vi "Ex6_Principal.vi"() -> ()   [LabVIEW 2019]
uses:
  Ex6_Secondaire.vi
panel:
  in  "stop":bool
  out "2D Picture":picture
  out "Max":i16
  out "Tentatives":i16
  in  "Ouvrir":bool
  out "Boolean 2":bool
  out "Boolean":bool
  in  "Knob 3":i8(knob) scale=0.0..9.0
  in  "Knob 2":i8(knob) scale=0.0..9.0
  in  "Knob":i16(knob) scale=0.0..9.0
  # "/"
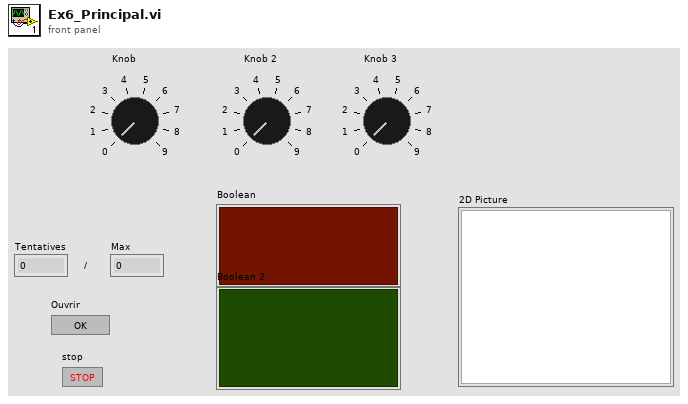
[diagram p1: front panel]
types:
  T1 = enum8{"Enabled", "Disabled", "Disabled and Grayed Out"}
  T2 = typedef "imagedata.ctl" = cluster{"image type":i32, "image depth":i32, "image":u8[], "mask":u8[], "colors":u32[], "Rectangle":cluster{"left":i16, "top":i16, "right":i16, "bottom":i16}}
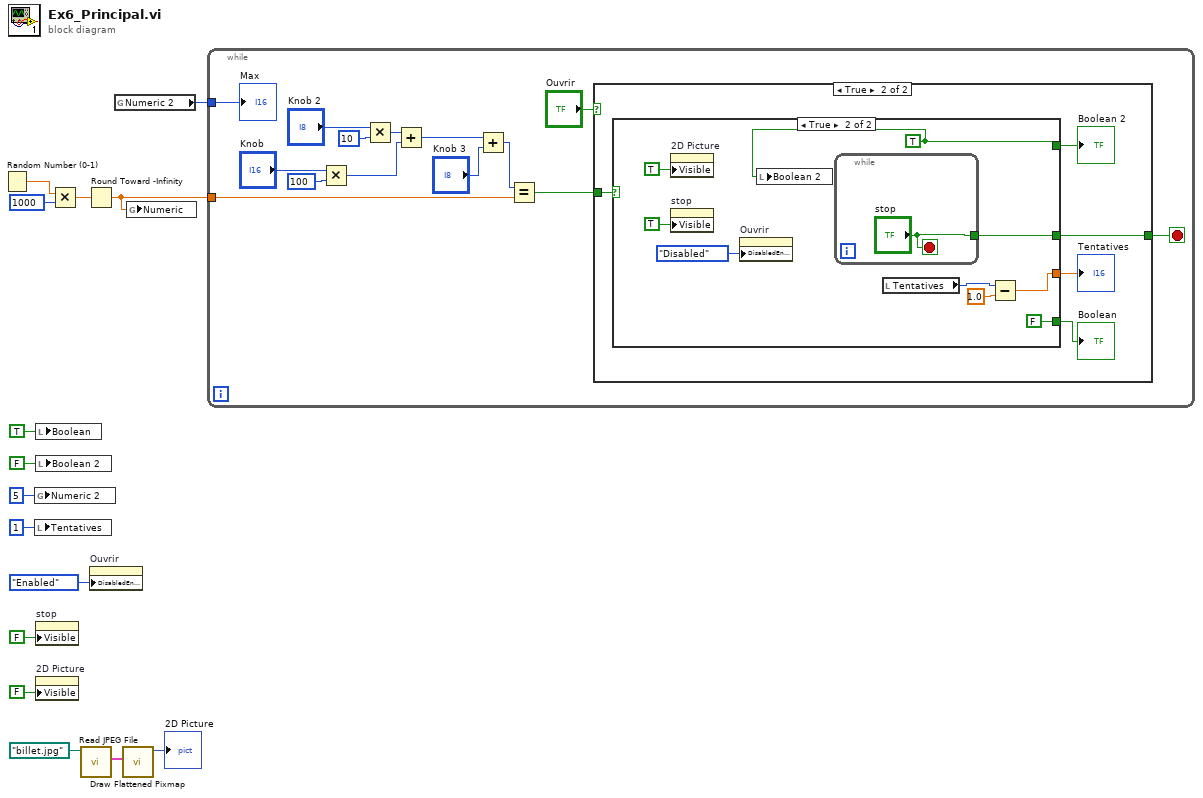
[diagram p0: block diagram]
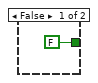
[diagram p2: hidden frame]
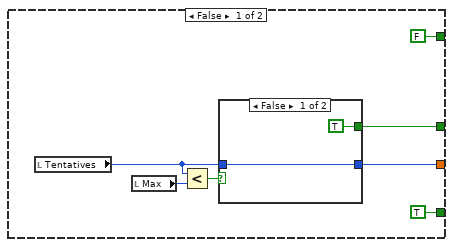
[diagram p3: hidden frame]
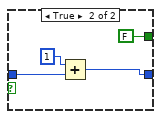
[diagram p4: hidden frame]
diagram:
  n1 = Random Number (0-1)() -> (number: 0 to 1=w15:dbl)
  n2 = global write "Ex6_Secondaire.vi" "Numeric 2"(i16 5 ("Numeric 2")) -> ()
  n3 = local write "Tentatives"(i8 1 ("Tentatives")) -> ()
  n4 = local write "Boolean"(TRUE) -> ()
  n5 = local write "Boolean 2"(FALSE) -> ()
  n6 = property on="stop" class="Bool"("Visible"=FALSE) -> ()  [unwired: 2 in, 2 out]
  n7 = property on="2D Picture" class="Pict"("Visible"=FALSE) -> ()  [unwired: 2 in, 2 out]
  n8 = Multiply(x=w15, y=1000 ("Numeric")) -> (x*y=w11:dbl)
  n9 = call <vilib>:"Read JPEG File.vi"("path to JPEG file"=path "billet.jpg") -> ("image data"=w5:T2)  [unwired: 8 in, 2 out]
  n10 = Round Toward -Infinity(1:w11) -> (0:w3:dbl)
  n11 = property on="Ouvrir" class="Bool"("DisabledEnum"=T1."Enabled" ("Disabled")) -> ()  [unwired: 2 in, 2 out]
  n12 = global read "Ex6_Secondaire.vi" "Numeric 2"() -> (w10:i16)
  n13 = call <vilib>:"Draw Flattened Pixmap.vi"("image data"=w5) -> ("new picture"=→"2D Picture":picture)  [unwired: 8 in]
  n14 = global write "Ex6_Secondaire.vi" "Numeric"(w3) -> ()
  n15 = while {
    tunnel: w3 -> [w18]
    tunnel: w10 -> [w17]
    stop <- w16 stop-if-true
    n16 = Multiply(x="Knob", y=i8 100) -> (x*y=w28:i16)
    n17 = Multiply(x="Knob 2", y=i8 10 ("x*y")) -> (x*y=w26:i8)
    n18 = Add(x=w26, y=w28) -> (x+y=w23:i16)
    n19 = Add(x=w23, y="Knob 3") -> (x+y=w20:i16)
    n20 = Equal?(x=w20, y=w18) -> (x = y?=w19:bool)
    n21 = case shown="True" "Ouvrir" {
      tunnel: w19 -> [_ w35]
      tunnel: [FALSE w31] -> w16
      frame False {
      }
      frame True {
        n22 = case shown="True" w35 {
          tunnel: [FALSE w49] -> w33
          tunnel: [TRUE FALSE] -> w34
          tunnel: [w38 w54] -> w32
          tunnel: [w36 w51] -> w31
          frame False {
            n23 = local read "Tentatives"() -> (w37:i16)
            n24 = local read "Max"() -> (w40:i16)
            n25 = Less?(x=w37, y=w40) -> (x < y?=w39:bool)
            n26 = case shown="False" w39 {
              tunnel: [w44 w47] -> w38
              tunnel: w37 -> [w44 w46]
              tunnel: [TRUE FALSE] -> w36
              frame False {
              }
              frame True {
                n27 = Add(x=i8 1, y=w46) -> (x+y=w47:i16)
              }
            }
          }
          frame True {
            w49 = TRUE
            n28 = property on="2D Picture" class="Pict"("Visible"=TRUE) -> ()  [unwired: 2 in, 2 out]
            n29 = property on="stop" class="Bool"("Visible"=TRUE) -> ()  [unwired: 2 in, 2 out]
            n30 = property on="Ouvrir" class="Bool"("DisabledEnum"=T1."Disabled" ("Disabled")) -> ()  [unwired: 2 in, 2 out]
            n31 = local write "Boolean 2"(w49) -> ()
            n32 = while {
              tunnel: ["stop"] -> w51
              stop <- "stop" stop-if-true
            }
            n33 = local read "Tentatives"() -> (w55:i16)
            n34 = Subtract(x=w55, y=1.0) -> (x-y=w54:dbl)
          }
        }
        "Boolean" <- w34
        "Boolean 2" <- w33
        "Tentatives" <- w32
      }
    }
    "Max" <- w17
  }
